vi "SerialCommunication.Initialize.vi"(8 "error in":errorcluster, 11 "Refnum In":refnum<vi>) -> (0 "error out":errorcluster, 3 "Refnum Out":refnum<vi>)   [LabVIEW 2020]
doc: "Initializes the library with a serial comport as the transport method"
uses:
  <vilib>/Instr/_visa.llb/VISA Configure Serial Port (Instr).vi
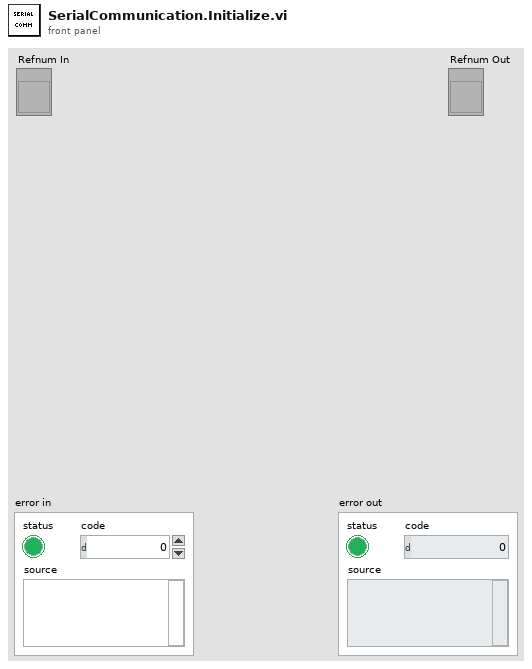
[diagram p1: front panel]
types:
  T1 = typedef "Parameters.ctl" = cluster{"Transport Parameters":T2, "Board Capabilities":map{i32, T4}}
  T2 = typedef "TransportParameters.ctl" = cluster{"Serial Communication":cluster{"Comport":refnum<visa-resource-name>, "No Response Timeout Ms":u32, "Response Complete Timeout Ms":u32, "Max Rx Length":u32, "Baud Rate":u32}, "Selected Transport":T3, "Initializer File Path":path, "Cleaner File Path":path, "Transporter File Path":path}
  T3 = typedef "SupportedTransports.ctl" = enum16{"Serial Communication Port"}
  T4 = typedef "FirmataPinCapabilitiesAndAnalogMapping.ctl" = cluster{"Supported Modes":T5[], "Analog Channel":u8}
  T5 = typedef "FirmataPinCapability.ctl" = cluster{"PinMode":T6, "Resolution":u8}
  T6 = typedef "FirmataClient.lvlib/FirmataPinModes.ctl" = enum16{"DigitalInput", "DigitalOutput", "AnalogInput", "PWM", "Servo", "Shift", "I2C", "OneWire", "Stepper", "Encoder", "Serial", "InputPullup", "Extended.SPI", "Extended.Sonar", "Extended.Tone", "Extended.DHT"}
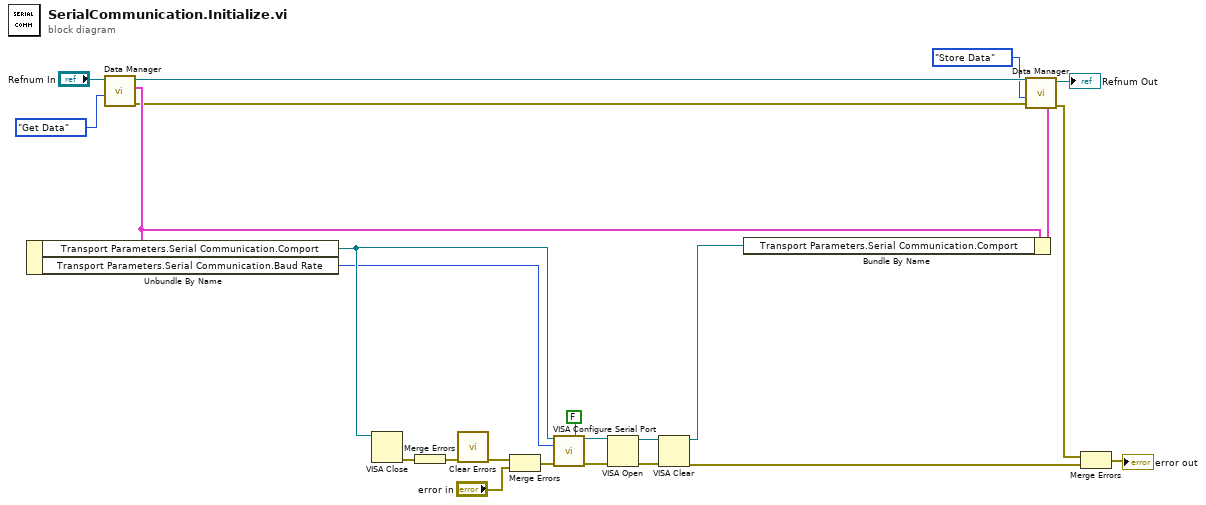
[diagram p0: block diagram]
diagram:
  n1 = call "Data Manager.vi"("Mode"=enum16{"Store Data", "Get Data", "Cleanup"}."Get Data", "Refnum In"="Refnum In") -> ("error out"=w16:errorcluster, "Data Out"=w21:T1, "Refnum Out"=w19:refnum<vi>)  [unwired: 7 in]
  n2 = Unbundle By Name(w21) -> ("Transport Parameters.Serial Communication.Comport"=w22:refnum<visa-resource-name>, "Transport Parameters.Serial Communication.Baud Rate"=w4:u32)
  n3 = VISA Close(VISA resource name=w22) -> (error out=w10:errorcluster)  [unwired: 1 in]
  n4 = Merge Errors(w10) -> (w9:errorcluster)
  n5 = call <vilib>:"Clear Errors.vi"("error in (no error)"=w9) -> ("error out"=w8:errorcluster)  [unwired: 5 in, 1 out]
  n6 = Merge Errors(w8, "error in") -> (w13:errorcluster)
  n7 = call-poly "VISA Configure Serial Port"("VISA resource name"=w22, "Enable Termination\nChar (T)"=FALSE ("Enable Termination\nChar (T)"), "baud rate (9600)"=w4, "error in (no error)"=w13) -> ("VISA resource name out"=w11:refnum<visa-resource-name>, "error out"=w12:errorcluster)  [unwired: 10 in]
  n8 = VISA Open(error in (no error)=w12, VISA resource name=w11) -> (VISA resource name=w6:refnum<visa-resource-name>, error out=w7:errorcluster)  [unwired: 3 in]
  n9 = VISA Clear(VISA resource name=w6, error in (no error)=w7) -> (VISA resource name out=w14:refnum<visa-resource-name>, error out=w1:errorcluster)
  n10 = Bundle By Name(cluster=w21, "Transport Parameters.Serial Communication.Comport"=w14) -> (w17:T1)
  n11 = call "Data Manager.vi"("error in (no error)"=w16, "Mode"=enum16{"Store Data", "Get Data", "Cleanup"}."Store Data", "Data In"=w17, "Refnum In"=w19) -> ("error out"=w3:errorcluster, "Refnum Out"=→"Refnum Out":refnum<vi>)  [unwired: 5 in, 1 out]
  n12 = Merge Errors(w3, w1) -> (→"error out":errorcluster)
